vi "PH_PSDBController.get Shot Types.vi"(0 "i ref in":refnum<vi>, 2 "possible Shot Types":T1[](array[typedef]), 5 "error IO":errorcluster) -> (14 "i ref out":refnum<vi>, 19 "error out":errorcluster)   [LabVIEW 2014, in "PH_PSDBController.lvlib"]
doc: "This VI sets the incoming possible shot IDs to own atributes, publishes them as DIM service and sets related to that the current shot ID."
uses:
  PH_PSDBController.lvlib
  User/Eisenbarth/psdb_lv/PSDB_Info.ctl
  CSCore/CSSystem/CoreLib/CoreLib.lvlib
  lib.lib/UtilityLib/UtilityLib.lvlib
  lib.lib/DimLVEvent/LVDimInterface/LVDimInterface.lvlib
  User/Eisenbarth/psdb_lv/PSDB.lvlib
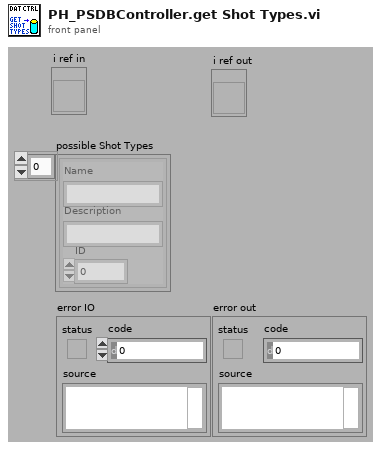
[diagram p1: front panel]
types:
  T1 = typedef "PSDB.lvlib/PSDB_Info.ctl" = cluster{"Name":string, "Description":string, "ID":i32}
  T2 = typedef "PH_PSDBController.lvlib/PH_PSDBController.i attribute.ctl" = cluster{"GUI Refs":cluster{"Data Status":refnum<vi>, "Current Shot ID":refnum<vi>, "active Subsystems":refnum<vi>, "Experiment Description":refnum<vi>, "Shot Comment":refnum<vi>, "Experiment":refnum<vi>, "Shottype":refnum<vi>, "Sequencer SM State":refnum<vi>, "Instances with Errors":refnum<vi>}, "Service ID Shot ID":i32, "Service ID wanted Subsystem":i32, "Data Status":T3, "Shotinformation":cluster{"Current Experiment ID":i32, "Current Shot Type":i32, "Current Comment":string}, "Data taking?":bool, "Service ID current Shottype":i32, "Service ID current Experiment":i32, "Service ID currentShot Comment":i32, "Service ID possible Shottypes":i32, "Service ID possible Experiments":i32, "possible Experiments":T1[], "possible Shottypes":T1[], "List":cluster{"Info":cluster{"Instance":string, "Data Status":T3}[], "GUI Ref":refnum<vi>, "Classname":string}[], "Subsystems Off?":cluster{"PHELIX_Beamline_fs_YLF_BL_Status":bool, "PHELIX_Beamline_ns_BL_Status":bool, "PHELIX_Beamline_PA_Input_BL_Status":bool, "PHELIX_Beamline_PA_MA_BL_Status":bool, "PHELIX_Beamline_MA_Z6_BL_Status":bool, "PHELIX_Beamline_MA_LB_BL_Status":bool, "PHELIX_Beamline_PA_LL_BL_Status":bool}, "PSDB Credentials":T4}
  T3 = typedef "PH_PSDBWriter.lvlib/PH_PSDBWriter.Data Status.ctl" = i16
  T4 = typedef "PH_Common.lvlib/PH_Connection.PSDB Credentials.ctl" = cluster{"PW":string, "ID":string, "DS":string}
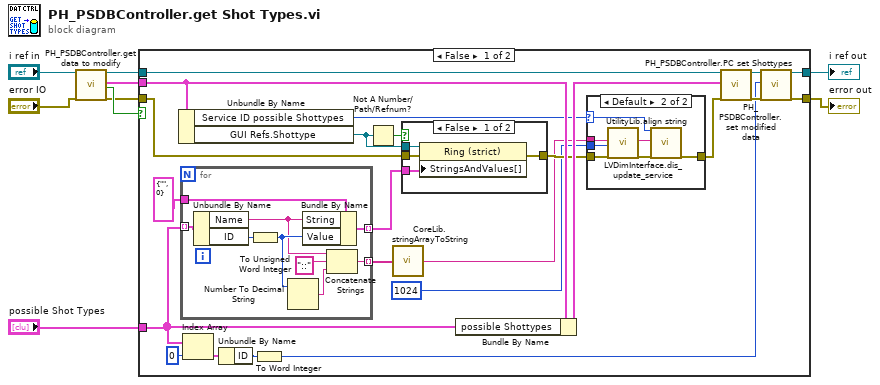
[diagram p0: block diagram]
diagram:
  n1 = call "PH_PSDBController.get data to modify.vi"("i ref in"="i ref in", "error in (no error)"="error IO") -> ("i ref out"=w4:refnum<vi>, "i attribute"=w3:T2, "timed out"=w9:bool, "error out"=w5:errorcluster)  [unwired: 14 in]
  n2 = case shown="False" w9 {
    tunnel: w3 -> [w24 _]
    tunnel: w4 -> [w22 w56]
    tunnel: w5 -> [w19 w55]
    tunnel: "possible Shot Types" -> [w17 _]
    tunnel: [w27 w56] -> w7
    tunnel: [w25 w55] -> w8
    frame False {
      n3 = Unbundle By Name(w24) -> ("Service ID possible Shottypes"=w12:i32, "GUI Refs.Shottype"=w21:refnum<vi>)
      n4 = for {
        tunnel: w17 -> [w49] mode=indexing
        tunnel: [w47] -> w16 mode=indexing
        tunnel: cluster{"String":string, "Value":u16} {"String"="", "Value"=0} -> [w46]
        tunnel: [w41] -> w15 mode=indexing
        n5 = Unbundle By Name(w49) -> ("Name"=w44:string, "ID"=w48:i32)
        n6 = To Unsigned Word Integer(number=w48) -> (unsigned 16bit integer=w45:u16)
        n7 = Number To Decimal String(number=w45) -> (decimal integer string=w42:string)  [unwired: 1 in]
        n8 = Bundle By Name(cluster=w46, "String"=w44, "Value"=w45) -> (w47:cluster{"String":string, "Value":u16})
        n9 = Concatenate Strings(w44, "::" ("string"), w42) -> (w41:string)
      }
      n10 = Index Array(array=w17, index=0 ("Exp ID")) -> (element=w31:T1)
      n11 = Unbundle By Name(w31) -> ("ID"=w30:i32)
      n12 = To Word Integer(number=w30) -> (16bit integer=w20:i16)
      n13 = Not A Number/Path/Refnum?(number/path/refnum=w21) -> (NaN/Path/Refnum?=w23:bool)
      n14 = call "CoreLib.stringArrayToString.vi"("Array"=w15) -> ("String"=w11:string)
      n15 = case shown="False" w23 {
        tunnel: w19 -> [w53 w54]
        tunnel: [w52 w54] -> w14
        tunnel: w21 -> [w51 _]
        tunnel: w16 -> [w50 _]
        frame False {
          n16 = property class="Ring (strict)"(reference=w51, error in=w53, "StringsAndValues[]"=w50) -> (error out=w52:errorcluster)  [unwired: 1 out]
        }
        frame True {
        }
      }
      n17 = Bundle By Name(cluster=w24, "possible Shottypes"=w17) -> (w29:T2)
      n18 = case shown="Default" w12 {
        selector: w12 -> [_ w34]
        tunnel: w14 -> [w33 w40]
        tunnel: w11 -> [_ w39]
        tunnel: u16 1024 ("stringLength (80)") -> [_ w38]
        tunnel: [w33 w36] -> w13
        frame -1 {
        }
        frame Default {
          n19 = call "UtilityLib.align string.vi"("stringIn"=w39, "stringLength (80)"=w38, "error in (no error)"=w40) -> ("stringOut"=w35:string, "error out"=w37:errorcluster)  [unwired: 15 in]
          n20 = call "LVDimInterface.dis_update_service.vi"("my_serviceID"=w34, "data"=w35, "error in (no error)"=w37) -> ("error out"=w36:errorcluster)  [unwired: 14 in, 2 out]
        }
      }
      n21 = call "PH_PSDBController.set modified data.vi"("i ref in"=w22, "i attribute"=w29, "error in (no error)"=w13) -> ("i ref out"=w28:refnum<vi>, "error out"=w26:errorcluster)  [unwired: 15 in]
      n22 = call "PH_PSDBController.PC set Shottypes.vi"("i ref in"=w28, "Shottype"=w20, "error IO"=w26) -> ("i ref out"=w27:refnum<vi>, "error out"=w25:errorcluster)  [unwired: 15 in]
    }
    frame True {
    }
  }
  "error out" <- w8
  "i ref out" <- w7
